vi "Fuzzy C-mean Clustering.vi"() -> ()   [LabVIEW 2011]
uses:
  <vilib>/Utility/file.llb/Write To Spreadsheet File (I64).vi
panel:
  out "tag":i32[](array[numeric])
  in  "군집_데이터_갯수":i32[](array[numeric])
  in  "파일(대화 상자 사용)":path
  out "initial_U0":ext[][](array[numeric])
  in  "cluster":i32=3
  out "Roop_Num":i32
  in  "임계값":ext=0.01
  out "Max":ext
  out "U0":ext[][](array[numeric])
  out "d":ext[][](array[numeric])
  out "v":ext[](array[numeric])
  out "n":i32
  out "j":i32
  out "U":ext[][](array[numeric])
  out "X":ext[][](array[numeric])
  # "Process"
  # "Option"
  # "Result"
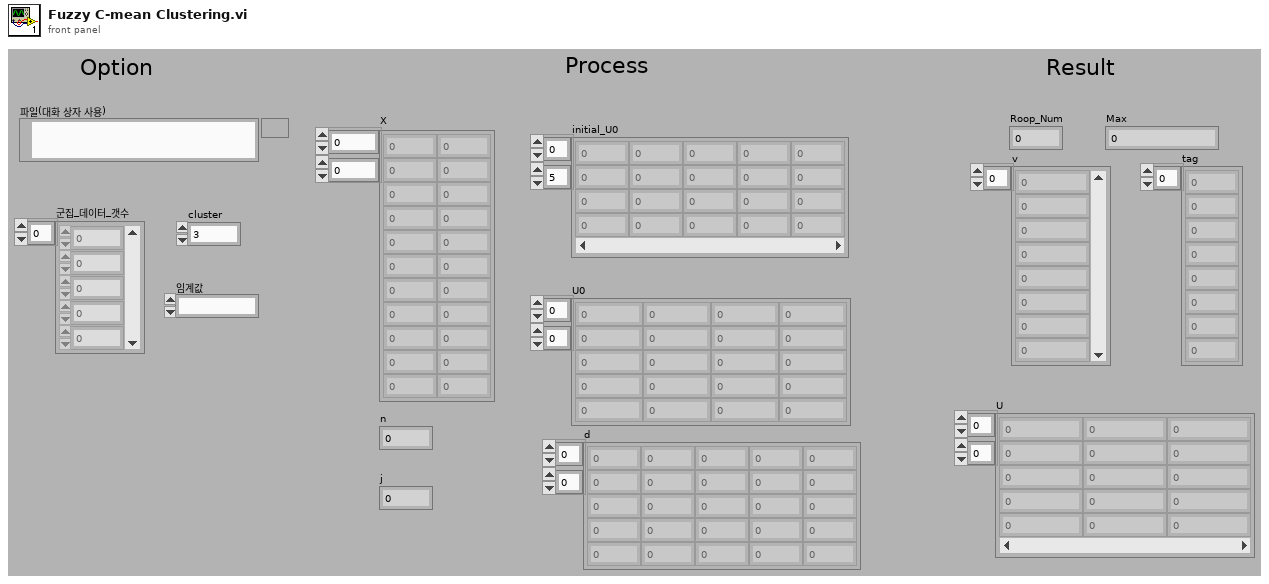
[diagram p1: front panel]
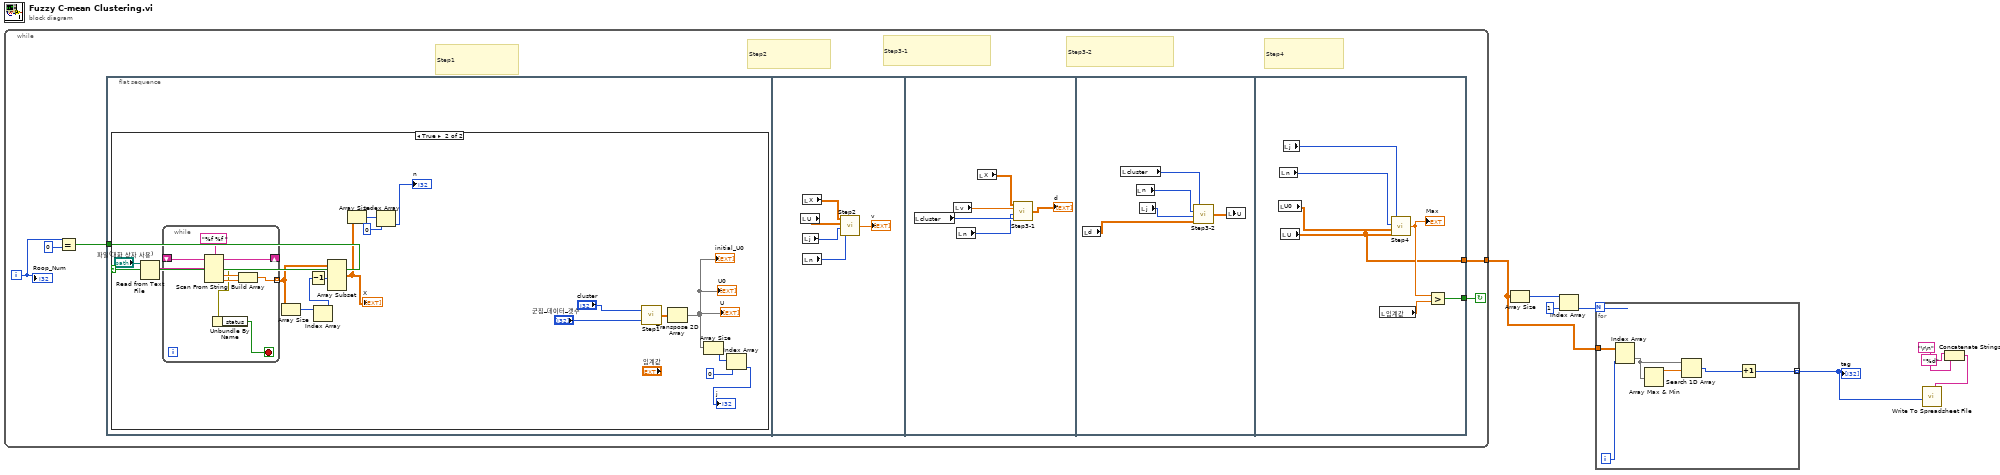
[diagram p0: block diagram]
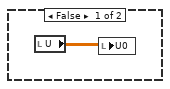
[diagram p2: hidden frame]
diagram:
  n1 = while {
    tunnel: [w9] -> w5
    i -> [w13]
    stop <- w11 continue-if-true
    # "Step4"
    # "Step3-2"
    # "Step3-1"
    # "Step2"
    # "Step1"
    n2 = Equal?(x=w13, y=0) -> (x = y?=w10:bool)
    n3 = flat-sequence {
      tunnel: w10 -> [w14]
      tunnel: [w58] -> w11
      tunnel: [w56] -> w9
      frame #0 {
        n4 = case shown="True" w14 {
          frame False {
            n5 = local read "U"() -> (w15:ext[][])
            n6 = local write "U0"(w15) -> ()
          }
          frame True {
            n7 = Read from Text File(file (use dialog)="파일(대화 상자 사용)") -> (text=w28:string)  [unwired: 3 in, 3 out]
            n8 = while {
              shift-right: [w39] -> _
              shift-left: w28 -> [w40]
              tunnel: [w35] -> w32 mode=indexing
              stop <- w33 stop-if-true
              n9 = Scan From String(format string="%f %f " ("포맷 문자열"), input string=w40) -> (remaining string=w39:string, error out=w34:errorcluster, output 1=w37:dbl, output 2=w36:dbl)  [unwired: 4 in, 1 out]
              n10 = Unbundle By Name(w34) -> ("status"=w33:bool)
              n11 = Build Array(w37, w36) -> (w35:dbl[])
            }
            n12 = Array Size(array=w32) -> (size(s)=w29:i32[])
            n13 = Index Array(array=w29) -> (element=w30:i32)  [unwired: 1 in]
            n14 = Decrement(x=w30) -> (x-1=w31:i32)
            n15 = Array Subset(array=w32, length (row)=w31) -> (w22:dbl[][])  [unwired: 3 in]
            "X" <- w22
            n16 = Array Size(array=w22) -> (size(s)=w25:i32[])
            n17 = Index Array(array=w25, index=0) -> (element=→"n":i32)
            n18 = call "Step1.vi"("군집_데이터"="군집_데이터_갯수", "클러스터"="cluster") -> ("ALL_U"=w19:ext[][])
            n19 = Transpose 2D Array(2D array=w19) -> (transposed array=w16:ext[][])
            "U" <- w16
            "U0" <- w16
            "initial_U0" <- w16
            n20 = Array Size(array=w16) -> (size(s)=w23:i32[])
            n21 = Index Array(array=w23, index=0) -> (element=→"j":i32)
          }
        }
      }
      frame #1 {
        n22 = local read "U"() -> (w43:ext[][])
        n23 = local read "X"() -> (w44:ext[][])
        n24 = local read "j"() -> (w41:i32)
        n25 = local read "n"() -> (w42:i32)
        n26 = call "Step2.vi"("n"=w42, "j"=w41, "U"=w43, "X"=w44) -> ("v"=→"v":dbl[])
      }
      frame #2 {
        n27 = local read "cluster"() -> (w50:i32)
        n28 = local read "v"() -> (w47:ext[])
        n29 = local read "n"() -> (w46:i32)
        n30 = local read "X"() -> (w48:ext[][])
        n31 = call "Step3-1.vi"("cluster"=w50, "n"=w46, "v"=w47, "X"=w48) -> ("Array"=→"d":dbl[][])
      }
      frame #3 {
        n32 = local read "d"() -> (w51:ext[][])
        n33 = local read "cluster"() -> (w54:i32)
        n34 = local read "n"() -> (w53:i32)
        n35 = local read "j"() -> (w52:i32)
        n36 = call "Step3-2.vi"("d"=w51, "j"=w52, "n"=w53, "cluster"=w54) -> ("Array"=w55:dbl[][])
        n37 = local write "U"(w55) -> ()
      }
      frame #4 {
        n38 = local read "U0"() -> (w61:ext[][])
        n39 = local read "n"() -> (w57:i32)
        n40 = local read "U"() -> (w56:ext[][])
        n41 = local read "j"() -> (w62:i32)
        n42 = local read "임계값"() -> (w59:ext)
        n43 = call "Step4.vi"("U"=w56, "U0"=w61, "n"=w57, "j"=w62) -> ("Numeric"=w60:dbl)
        "Max" <- w60
        n44 = Greater?(x=w60, y=w59) -> (0:w58:bool)
      }
    }
    "Roop_Num" <- w13
  }
  n45 = Array Size(array=w5) -> (size(s)=w8:i32[])
  n46 = Index Array(array=w8, index=1) -> (element=w6:i32)
  n47 = for {
    N: w6 -> [_]
    tunnel: w5 -> [w68]
    tunnel: [w63] -> w1 mode=indexing
    i -> [w67]
    n48 = Index Array(array=w68, index (col)=w67) -> (element=w66:ext[])  [unwired: 1 in]
    n49 = Array Max & Min(array=w66) -> (max value=w65:ext)  [unwired: 3 out]
    n50 = Search 1D Array(1D array=w66, element=w65) -> (index of element=w64:i32)  [unwired: 1 in]
    n51 = Increment(x=w64) -> (x+1=w63:i32)
  }
  "tag" <- w1
  n52 = Concatenate Strings("%d" ("format (%d)"), "\r\n") -> (w2:string)
  n53 = call-poly <vilib>:"Write To Spreadsheet File.vi"("format (%d)"=w2, "1D data"=w1) -> ()  [unwired: 6 in, 1 out]
